vi "Read Array of Active Task.vi"(8 "error in (no error)":errorcluster, 11 "National Instrument USB-6501 in":refnum<class "National Instrument USB-6501.lvclass">) -> (0 "error out":errorcluster, 2 "Array of Active Task":T1(array[cluster]), 3 "National Instrument USB-6501 out":refnum<class "National Instrument USB-6501.lvclass">)   [LabVIEW 2014, in "Generic Data Acquisition.lvlib" / "National Instrument USB-6501.lvlib" / "National Instrument USB-6501.lvclass"]
uses:
  National Instrument USB-6501.lvclass
  National Instrument USB-6501.lvclass/National Instrument USB-6501.ctl
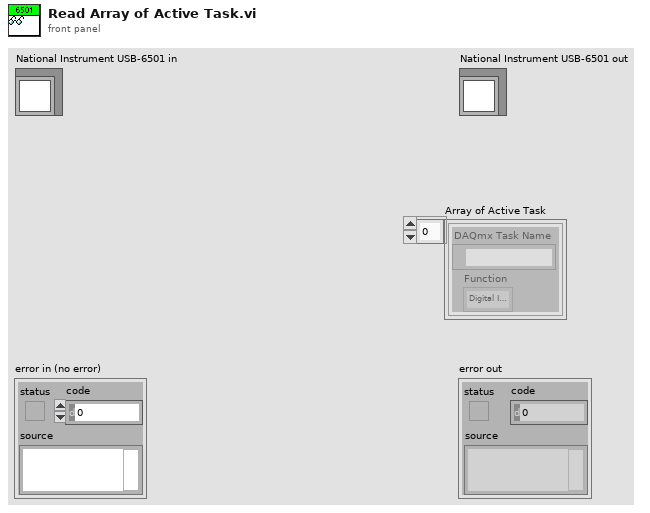
[diagram p1: front panel]
types:
  T1 = cluster{"DAQmx Task Name":refnum<k21>, "Function":enum16{"Digital Input", "Digital Output"}}[]
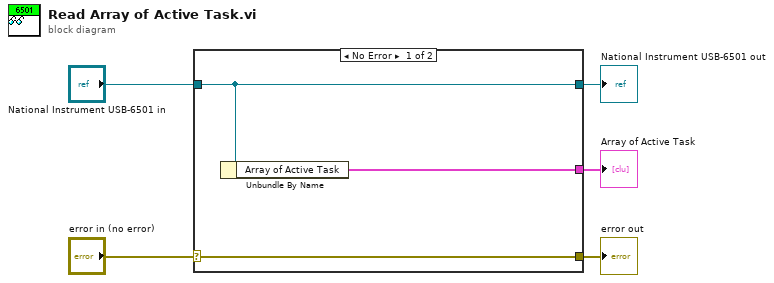
[diagram p0: block diagram]
diagram:
  n1 = case shown="No Error" "error in (no error)" {
    selector: "error in (no error)" -> [w8 w9]
    tunnel: [w8 w9] -> w4
    tunnel: [w7 w10] -> w2
    tunnel: "National Instrument USB-6501 in" -> [w7 w10]
    tunnel: [w6 _] -> w1
    frame No Error {
      n2 = Unbundle By Name(w7) -> ("Array of Active Task"=w6:T1)
    }
    frame Error {
    }
  }
  "error out" <- w4
  "National Instrument USB-6501 out" <- w2
  "Array of Active Task" <- w1
